vi "Test Save C-scan.vi"() -> ()   [LabVIEW 2018]
panel:
  out "size(s)":i32[](array[numeric])
  in  "stop":bool
  out "time":dbl
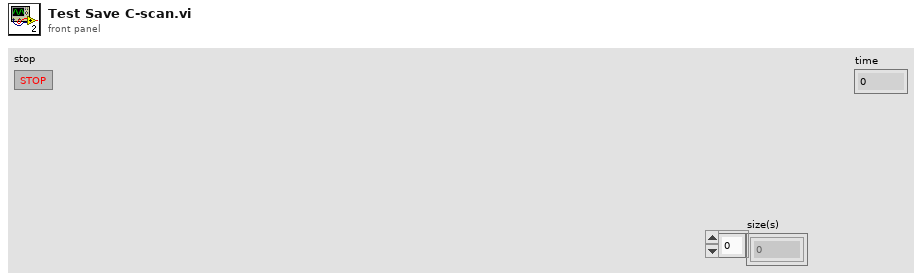
[diagram p1: front panel]
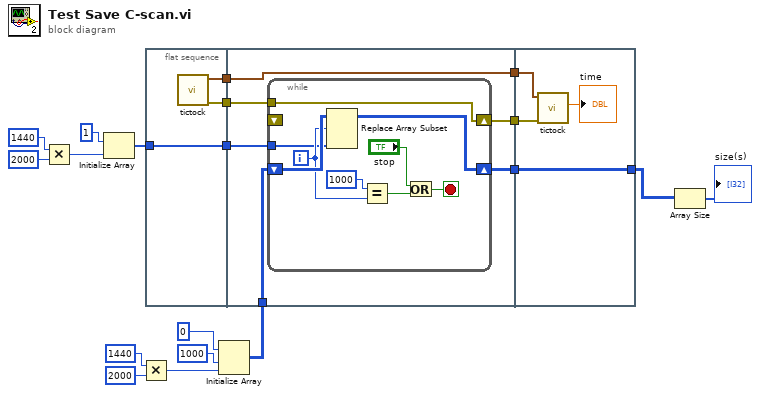
[diagram p0: block diagram]
diagram:
  n1 = Multiply(x=u32 1440 ("element"), y=u32 2000 ("element")) -> (x*y=w6:u32)
  n2 = Initialize Array(u16 1 ("element"), w6) -> (w16:u16[])
  n3 = Multiply(x=u32 1440 ("element"), y=u32 2000 ("element")) -> (x*y=w3:u32)
  n4 = flat-sequence {
    tunnel: w16 -> [w20]
    tunnel: [w20] -> w15
    tunnel: [w22] -> w13
    tunnel: [w21] -> w12
    tunnel: w15 -> [w28]
    tunnel: [w27] -> w14
    tunnel: w13 -> [w27]
    tunnel: w12 -> [w26]
    tunnel: [w25] -> w11
    tunnel: w7 -> [w24]
    tunnel: [w23] -> w5
    tunnel: w14 -> [w41]
    tunnel: w11 -> [w40]
    tunnel: w5 -> [w38]
    tunnel: [w38] -> w1
    frame #0 {
      n5 = call "tictock.vi"() -> ("error out"=w21:errorcluster, "seconds since 1Jan1904"=w22:timestamp)  [unwired: 9 in, 1 out]
    }
    frame #1 {
      n6 = while {
        tunnel: w28 -> [w29]
        tunnel: w26 -> [w36]
        shift-right: [w36] -> w25
        shift-left: _ -> [_]
        shift-right: [w31] -> w23
        shift-left: w24 -> [w32]
        i -> [w30]
        stop <- w34 stop-if-true
        n7 = Replace Array Subset(array=w32, new element=w29, index (row)=w30) -> (w31:u16[][])  [unwired: 1 in]
        n8 = Equal?(x=1000, y=w30) -> (x = y?=w35:bool)
        n9 = Or(x="stop", y=w35) -> (x .or. y?=w34:bool)
      }
    }
    frame #2 {
      n10 = call "tictock.vi"("error in (no error)"=w40, "seconds since 1Jan1904 2"=w41) -> ("Numeric"=→"time":dbl)  [unwired: 7 in, 2 out]
    }
  }
  n11 = Initialize Array(u16 0 ("element"), 1000 ("dimension size"), w3) -> (w7:u16[][])
  n12 = Array Size(array=w1) -> (size(s)=→"size(s)":i32[])
